vi "exnSpectralBlock mod exp dyn x attribs 1signal.vi"(8 "error in (no error)":errorcluster, 11 "waveform in":waveform(dbl)) -> (0 "error out":errorcluster, 3 "waveform out":waveform(dbl))   [LabVIEW 2017]
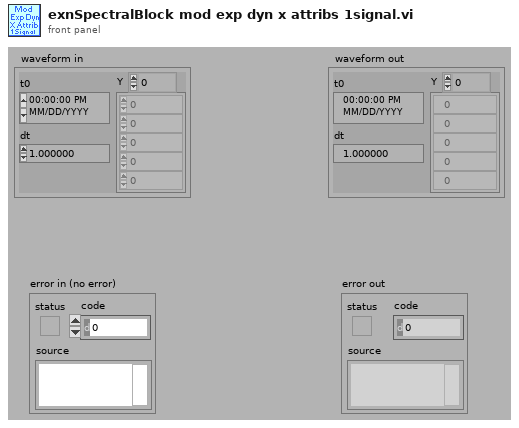
[diagram p1: front panel]
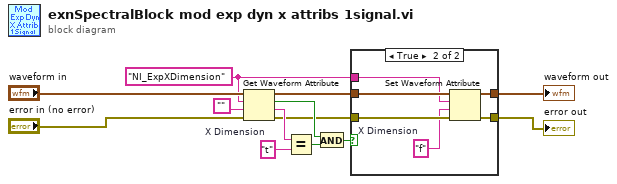
[diagram p0: block diagram]
diagram:
  w6 = "t"  # X Dimension
  w9 = "NI_ExpXDimension" ("name")
  n1 = Get Waveform Attribute(4:"error in (no error)", 5:"", 6:w9, 7:"waveform in") -> (0:w2:errorcluster, 1:w8:string, 2:w3:bool, 3:w1:waveform(dbl))
  n2 = Equal?(x=w8, y=w6) -> (x = y?=w4:bool)
  n3 = And(x=w3, y=w4) -> (x .and. y?=w7:bool)
  n4 = case shown="True" w7 {
    tunnel: w1 -> [w15 w21]
    tunnel: w2 -> [w14 w20]
    tunnel: [w14 w19] -> w12
    tunnel: [w15 w18] -> w11
    tunnel: w9 -> [_ w17]
    frame False {
    }
    frame True {
      w16 = "f"  # X Dimension
      n5 = Set Waveform Attribute(4:w20, 5:w16, 6:w17, 7:w21) -> (0:w19:errorcluster, 3:w18:waveform(dbl))  [unwired: 1 out]
    }
  }
  "error out" <- w12
  "waveform out" <- w11
